vi "AMC Dispatch PingAll.vi"(7 "IgnoreSender (T)":bool=TRUE, 8 "error in (no error)":errorcluster, 9 "Timeout (1000 ms)":i32=1000) -> (0 "error out":errorcluster, 2 "Response":string, 3 "Messages":T1[](array[typedef]))   [LabVIEW 2017]
uses:
  Tools/Keyed Array/Tools_KeyedArray KeyedArray.ctl
  subVIs/TypeDefs/amc_Message.ctl
  subVIs/amc_Globals.vi
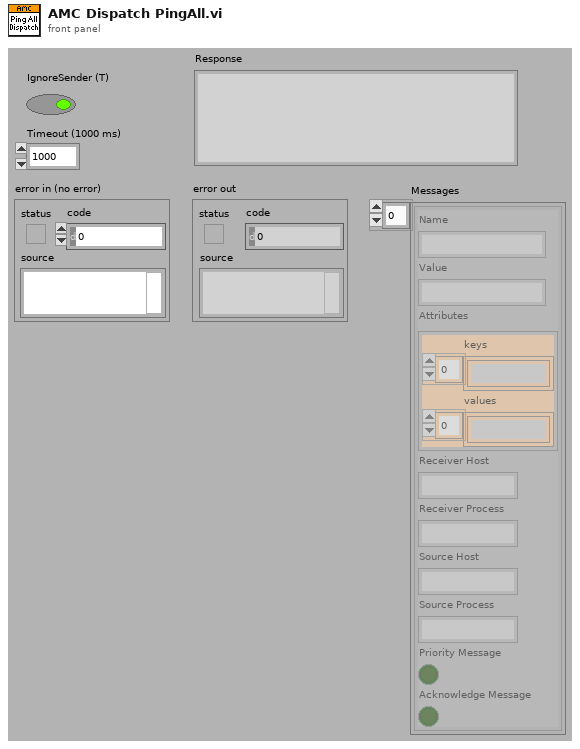
[diagram p1: front panel]
types:
  T1 = typedef "amc_Message.ctl" = cluster{"Name":string, "Value":string, "Attributes":T2, "Receiver Host":string, "Receiver Process":string, "Source Host":string, "Source Process":string, "Priority Message":bool, "Acknowledge Message":bool}
  T2 = typedef "Tools_KeyedArray KeyedArray.ctl" = cluster{"keys":string[], "values":string[]}
  T3 = typedef "amc_Message Queue.ctl" = refnum<queue>
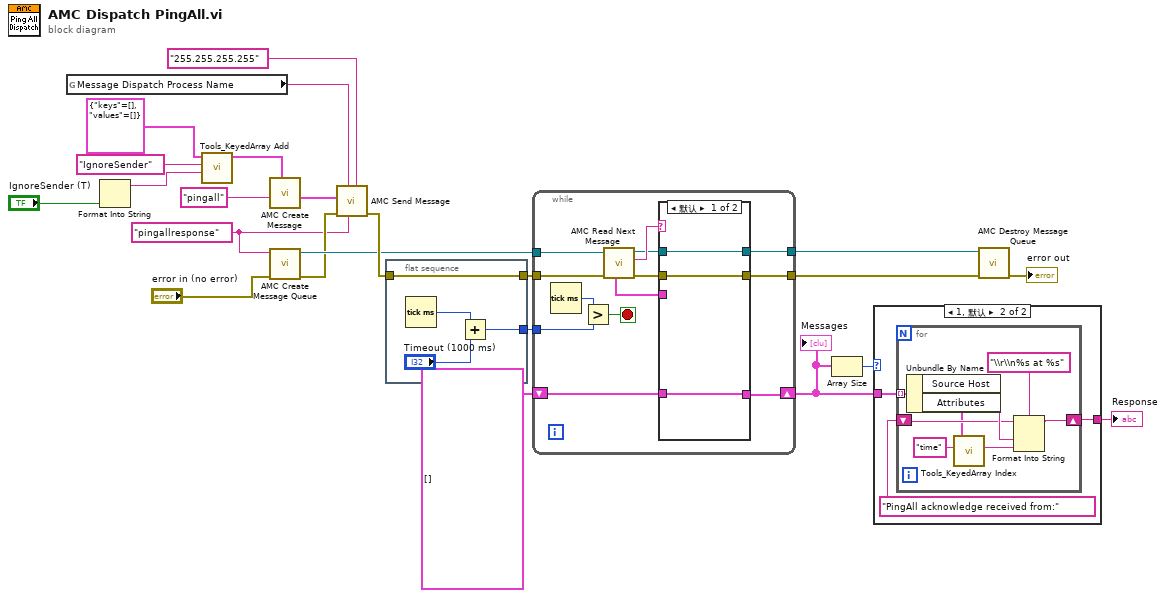
[diagram p0: block diagram]
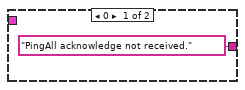
[diagram p2: hidden frame]
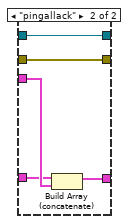
[diagram p3: hidden frame]
diagram:
  w3 = "pingallresponse" ("message queue name")
  n1 = global read "amc_Globals.vi" "Message Dispatch Process Name"() -> (w2:string)
  n2 = Format Into String("IgnoreSender (T)") -> (resulting string=w4:string)  [unwired: 3 in, 1 out]
  n3 = call "Tools_KeyedArray Add.vi"("value"=w4, "key"="IgnoreSender", "array in"=T2 {"keys"=[], "values"=[]}) -> ("array out"=w8:T2)  [unwired: 1 in, 3 out]
  n4 = call "AMC Create Message.vi"("Attributes"=w8, "Name"="pingall") -> ("Message"=w9:T1)  [unwired: 1 in, 8 out]
  n5 = call "AMC Create Message Queue.vi"("error in (no error)"="error in (no error)", "Message Queue Name"=w3) -> ("error out"=w15:errorcluster, "Message Queue out"=w16:T3)  [unwired: 2 in, 6 out]
  n6 = call "AMC Send Message.vi"("Receiver Host"="255.255.255.255" ("receiver host"), "Source Process"=w3, "Receiver Process"=w2, "error in (no error)"=w15, "Message"=w9) -> ("error out"=w21:errorcluster)  [unwired: 3 in, 3 out]
  n7 = flat-sequence {
    tunnel: [w27] -> w20
    tunnel: w21 -> [w27]
    tunnel: [w24] -> w19
    frame #0 {
      n8 = Tick Count (ms)() -> (millisecond timer value=w26:u32)
      n9 = Add(x=w26, y="Timeout (1000 ms)") -> (x+y=w24:u32)
    }
  }
  n10 = while {
    tunnel: w20 -> [w40]
    tunnel: [w35] -> w17
    tunnel: [w34] -> w18
    tunnel: w16 -> [w33]
    tunnel: w19 -> [w31]
    shift-right: [w30] -> w11
    shift-left: T1[] [] -> [w29]
    stop <- w28 stop-if-true
    n11 = Tick Count (ms)() -> (millisecond timer value=w32:u32)
    n12 = Greater?(x=w32, y=w31) -> (0:w28:bool)
    n13 = call "AMC Read Next Message.vi"("error in (no error)"=w40, "Message Queue in"=w33) -> ("error out"=w37:errorcluster, "Message Name"=w39:string, "Message Queue out"=w36:T3, "Message"=w38:T1)  [unwired: 2 in, 4 out]
    n14 = case shown="默认" w39 {
      tunnel: w38 -> [_ w45]
      tunnel: [w41 w46] -> w30
      tunnel: [w42 w48] -> w35
      tunnel: w37 -> [w42 w48]
      tunnel: [w43 w47] -> w34
      tunnel: w36 -> [w43 w47]
      tunnel: w29 -> [w41 w44]
      frame Default {
      }
      frame "pingallack" {
        n15 = Build Array (concatenate)(w44, w45) -> (w46:T1[])
      }
    }
  }
  "Messages" <- w11
  n16 = Array Size(array=w11) -> (size(s)=w13:i32)
  n17 = case shown="1, 默认" w13 {
    tunnel: ["PingAll acknowledge not received." w50] -> w12
    tunnel: w11 -> [_ w52]
    frame 0 {
    }
    frame 1, Default {
      n18 = for {
        shift-right: [w57] -> w50
        shift-left: "PingAll acknowledge received from:" ("format string") -> [w56]
        tunnel: w52 -> [w58] mode=indexing
        n19 = Unbundle By Name(w58) -> ("Source Host"=w60:string, "Attributes"=w54:T2)
        n20 = call "Tools_KeyedArray Index.vi"("key"="time", "array in"=w54) -> ("value"=w53:string)  [unwired: 2 in, 3 out]
        n21 = Format Into String(format string="\\r\\n%s at %s", initial string=w56, w60, w53) -> (resulting string=w57:string)  [unwired: 1 in, 1 out]
      }
    }
  }
  "Response" <- w12
  n22 = call "AMC Destroy Message Queue.vi"("error in (no error)"=w17, "Message Queue in"=w18) -> ("error out"=→"error out":errorcluster)  [unwired: 9 out]
